vi "Group Count.vi"(8 "error in (no error)":errorcluster, 11 "Plugin Configuration in":refnum<class "Plugin Configuration.lvclass">) -> (0 "error out":errorcluster, 2 "group count":i32, 3 "Plugin Configuration out":refnum<class "Plugin Configuration.lvclass">)   [LabVIEW 2019, in "DSF Core.lvlib" / "Plugin Configuration.lvclass"]
uses:
  Plugin Configuration.lvclass
  Plugin Configuration.lvclass/Plugin Configuration.ctl
  Thread/Thread Configuration.lvclass
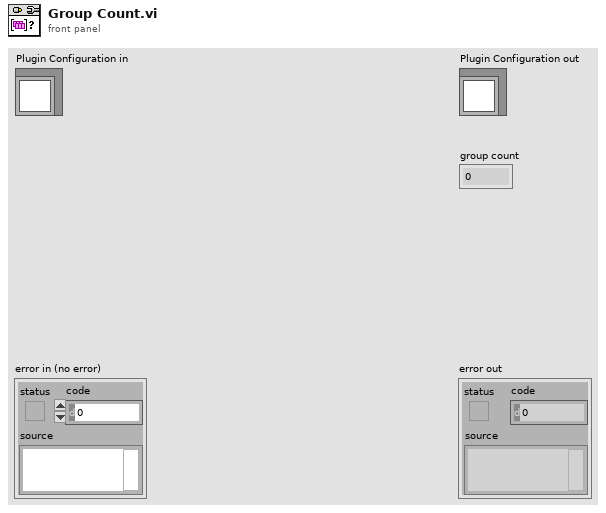
[diagram p1: front panel]
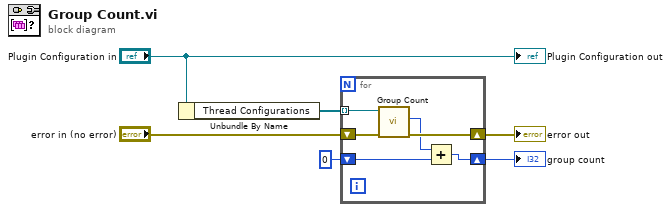
[diagram p0: block diagram]
diagram:
  n1 = Unbundle By Name("Plugin Configuration in") -> ("Thread Configurations"=w5:refnum<class "Thread Configuration.lvclass">[])
  n2 = for {
    tunnel: w5 -> [w12] mode=indexing
    shift-right: [w11] -> w3
    shift-left: "error in (no error)" -> [w10]
    shift-right: [w9] -> w1
    shift-left: 0 -> [w8]
    n3 = call-dynamic "Group Count.vi"("error in (no error)"=w10, "Thread Configuration in"=w12) -> ("error out"=w11:errorcluster, "group count"=w7:i32)  [unwired: 7 in, 1 out]
    n4 = Add(x=w7, y=w8) -> (x+y=w9:i32)
  }
  "error out" <- w3
  "group count" <- w1
  "Plugin Configuration out" <- "Plugin Configuration in"
